vi "GetSampleData.vi"(8 "错误输入（无错误）":errorcluster, 11 "SampleInfoTime":string) -> (0 "错误输出":errorcluster, 1 "是否存在记录":bool, 2 "记录数":i32, 3 "所有记录":string[][](array[string]))   [LabVIEW 2014, in "cyy.lvlib"]
uses:
  CYY/cyy.lvlib
  DataBase.lvlib
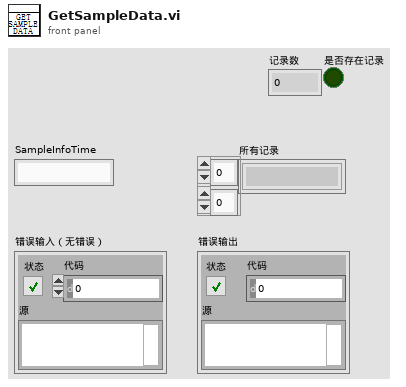
[diagram p1: front panel]
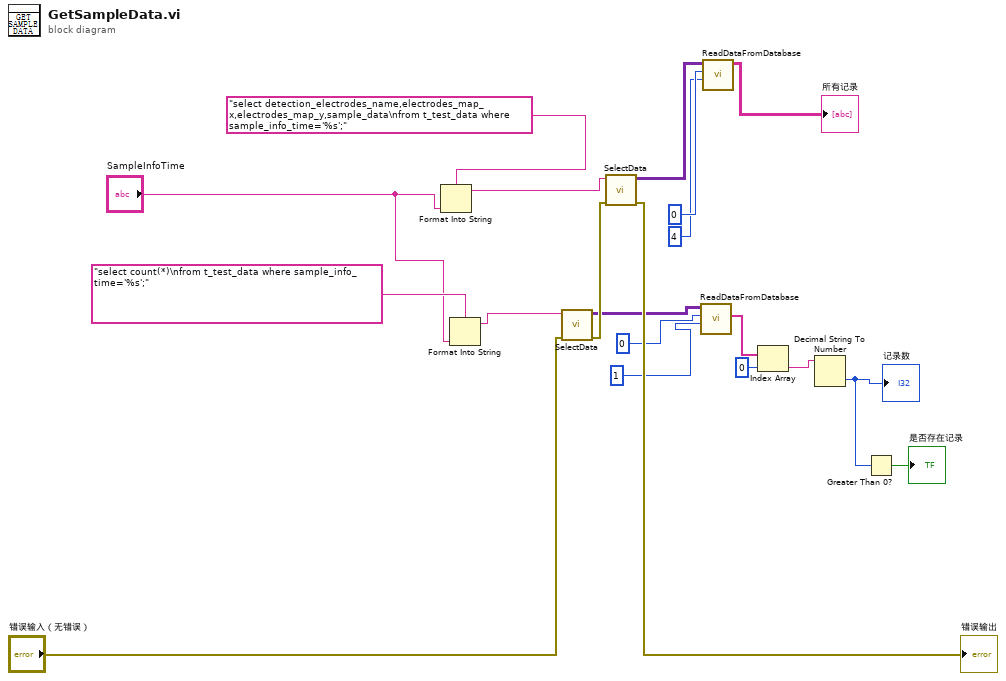
[diagram p0: block diagram]
diagram:
  n1 = Format Into String(format string="select detection_electrodes_name,electrodes_map_x,electrodes_map_y,sample_data\nfrom t_test_data where sample_info_time='%s';", "SampleInfoTime") -> (resulting string=w18:string)  [unwired: 2 in, 1 out]
  n2 = Format Into String(format string="select count(*)\nfrom t_test_data where sample_info_time='%s';", "SampleInfoTime") -> (resulting string=w15:string)  [unwired: 2 in, 1 out]
  n3 = call "SelectData.vi"("SQL query"=w15, "error in"="错误输入（无错误）") -> ("recordset data"=w4:variant[][], "error out"=w14:errorcluster)  [unwired: 6 in]
  n4 = call "SelectData.vi"("SQL query"=w18, "error in"=w14) -> ("recordset data"=w8:variant[][], "error out"=→"错误输出":errorcluster)  [unwired: 6 in]
  n5 = call "ReadDataFromDatabase.vi"("长度"=1, "index"=0, "recordset data"=w4) -> ("一行记录"=w1:string[])  [unwired: 7 in, 1 out]
  n6 = call "ReadDataFromDatabase.vi"("长度"=4, "index"=0, "recordset data"=w8) -> ("所有记录"=→"所有记录":string[][])  [unwired: 7 in, 1 out]
  n7 = Index Array(array=w1, index=0 ("索引")) -> (element=w11:string)
  n8 = Decimal String To Number(string=w11) -> (number=w10:i32)  [unwired: 2 in, 1 out]
  "记录数" <- w10
  n9 = Greater Than 0?(x=w10) -> (x > 0?=→"是否存在记录":bool)
